vi "Acquire Data using 5772 without DRAM_sim.vi"() -> ()   [LabVIEW 2011]
uses:
  <vilib>/Platform/TimedLoop/XDataNode/timing_clust.ctl
  <vilib>/Platform/TimedLoop/XDataNode/nitl_modes.ctl
  <vilib>/Platform/TimedLoop/XDataNode/wakeup.ctl
  Channel Data/Data from Channel 0 and Channel 1.vi
  <instrlib>/FlexRIO/Libraries/Acquisition Engine/FPGA/Implementation/acqEngineNRecordStateMachine.vi
  <vilib>/rvi/FIFO/Fifo_Resource/nirvififoEmulationSetSize.vi
  <vilib>/rvi/DataTransferAndStorage/Container/Common/niFpgaContainerGetUniqueNameForEmu.vi
  <instrlib>/FlexRIO/Libraries/Acquisition Engine/FPGA/Implementation/Pack 8-I16 As U128.vi
  <instrlib>/FlexRIO/Libraries/Host Transfer/FPGA/Implementation/Write to Host-Bound Domain (128-bit to 64-bit).vi
  <vilib>/Platform/TimedLoop/XDataNode/XDataNode.xnode
  <vilib>/rvi/FXPMathLib/basic elements/FxpDiscreteDelay/XNode/nifxpmath_DiscreteDelay.xnode
  <vilib>/rvi/DataTransferAndStorage/Container/XNode/niFpgaContainer.xnode
  <vilib>/rvi/FIFO/Fifo_Resource/nirvififoEmulationWrite.vi
  <vilib>/rvi/FIFO/Fifo_Resource/nirvififoEmulationRead.vi
  <vilib>/Platform/TimedLoop/XDataNode/XDNodeRunTimeDep.lvlib
  <vilib>/eio/EIONode/EIONode.xnode
  <instrlib>/FlexRIO/Libraries/Acquisition Engine/Acquisition Engine.lvlib
  <vilib>/rvi/eio/common/nirviEmuTemplateMethod_errors.vi
  <instrlib>/FlexRIO/Libraries/Host Transfer/Host Transfer.lvlib
panel:
  out "Channel 1":i16(graph)
  out "Channel 0":i16(graph)
  out "NumSamplestoHost":u32
  out "NumSamplesAcquired":u32
  out "Host FIFO Timed Out?":bool
  in  "Host Trigger":bool=TRUE
  in  "Trigger Type":T1(ring)=enum."Software Trigger"
  out "IO Module\\Initialization Done":bool
  in  "acq.Post Trig":u32=10
  in  "acq.Pre Trig":u32=2 min=2 step=1
  in  "acq.Record Count":u32=1
  in  "acq.Initiate":bool=TRUE
  # "Digitial Trigger Input:\nPXI_Trig0 or DIO 0 on CB Front Panel"
  # "Interactive Mode Instructions\n1) Run the Emulation Mode VI for Stimulus\n1) Click on acq.Initiate, First to False and Then to True\n2) Click on Host Trigger"
  # "Trigger Selection"
  # "Acquisition Engine"
  # "Status"
  # "Record Retrieval"
  # "Memory Configuration"
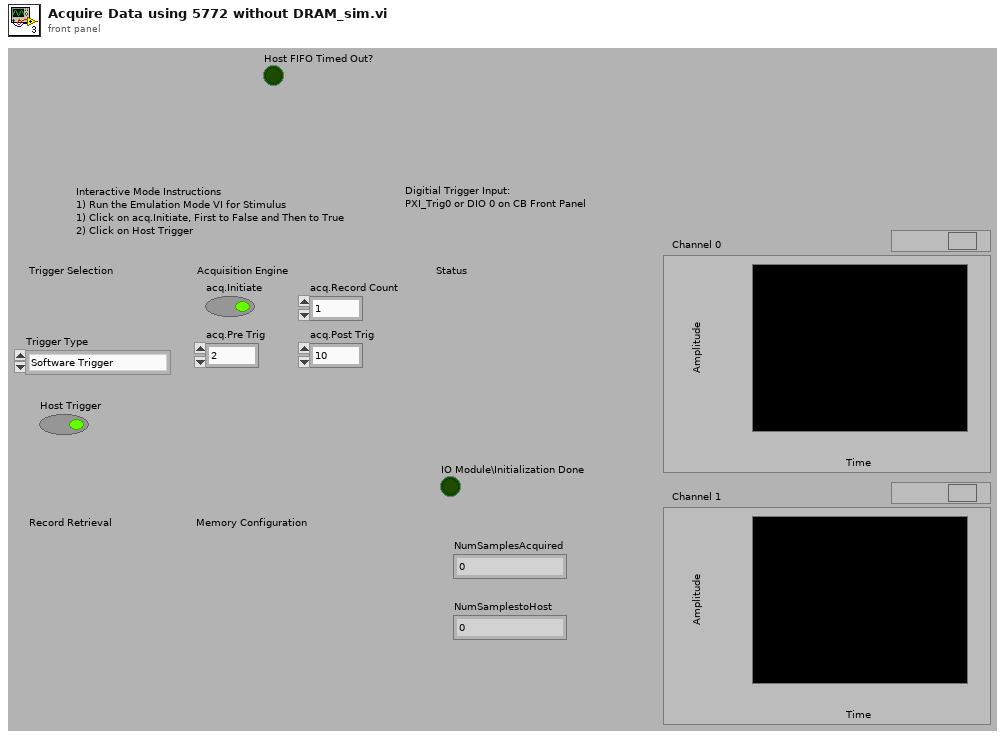
[diagram p1: front panel]
types:
  T1 = enum8{"Immediate Trigger", "Software Trigger", "External Digital Trigger", "Analog Trigger"}
  T2 = typedef "XDNodeRunTimeDep.lvlib/timing_clust.ctl" = cluster{"Expected End [f-1]":u64, "Actual End [f-1]":u64, "Finished Late? [f-1]":bool, "Expected End [i-1]":u64, "Actual End [i-1]":u64, "Finished Late? [i-1]":bool, "Expected Start [i]":u64, "Actual Start [i]":u64, "Expected Start [f]":u64, "Actual Start [f]":u64, "Source Name":string, "Structure Name":string, "Period":i64, "Deadline":i64, "Offset":i64, "Start":i64, "Priority":i32, "Timeout":i32, "Mode":T3, "Wakeup Reason":T4, "Error":errorcluster, "Source Type":string, "Secondary Source Type":string, "Global End Time":u64, "Global Start Time":u64, "Frame Duration":u64, "Iteration Duration":u64, "Assigned CPU":i32, "I/O Scan Engine Mode":u32}
  T3 = typedef "XDNodeRunTimeDep.lvlib/nitl_modes.ctl" = enum32{"No Change", "Process missed periods, maintain original phase", "Discard missed periods, maintain original phase", "Process missed periods, ignore original phase", "Discard missed periods, ignore original phase"}
  T4 = typedef "XDNodeRunTimeDep.lvlib/wakeup.ctl" = enum32{"Normal", "Aborted", "Asynchronous wakeup", "Timing source error", "Timed loop error", "Timeout"}
  T5 = typedef "Memory.lvlib/U128.ctl" = u8[]
  T6 = typedef "acqEngineStates v1.ctl" = cluster{"Triggered":bool, "TrigArmed":bool, "RdyForArm":bool, "Reserved":bool}
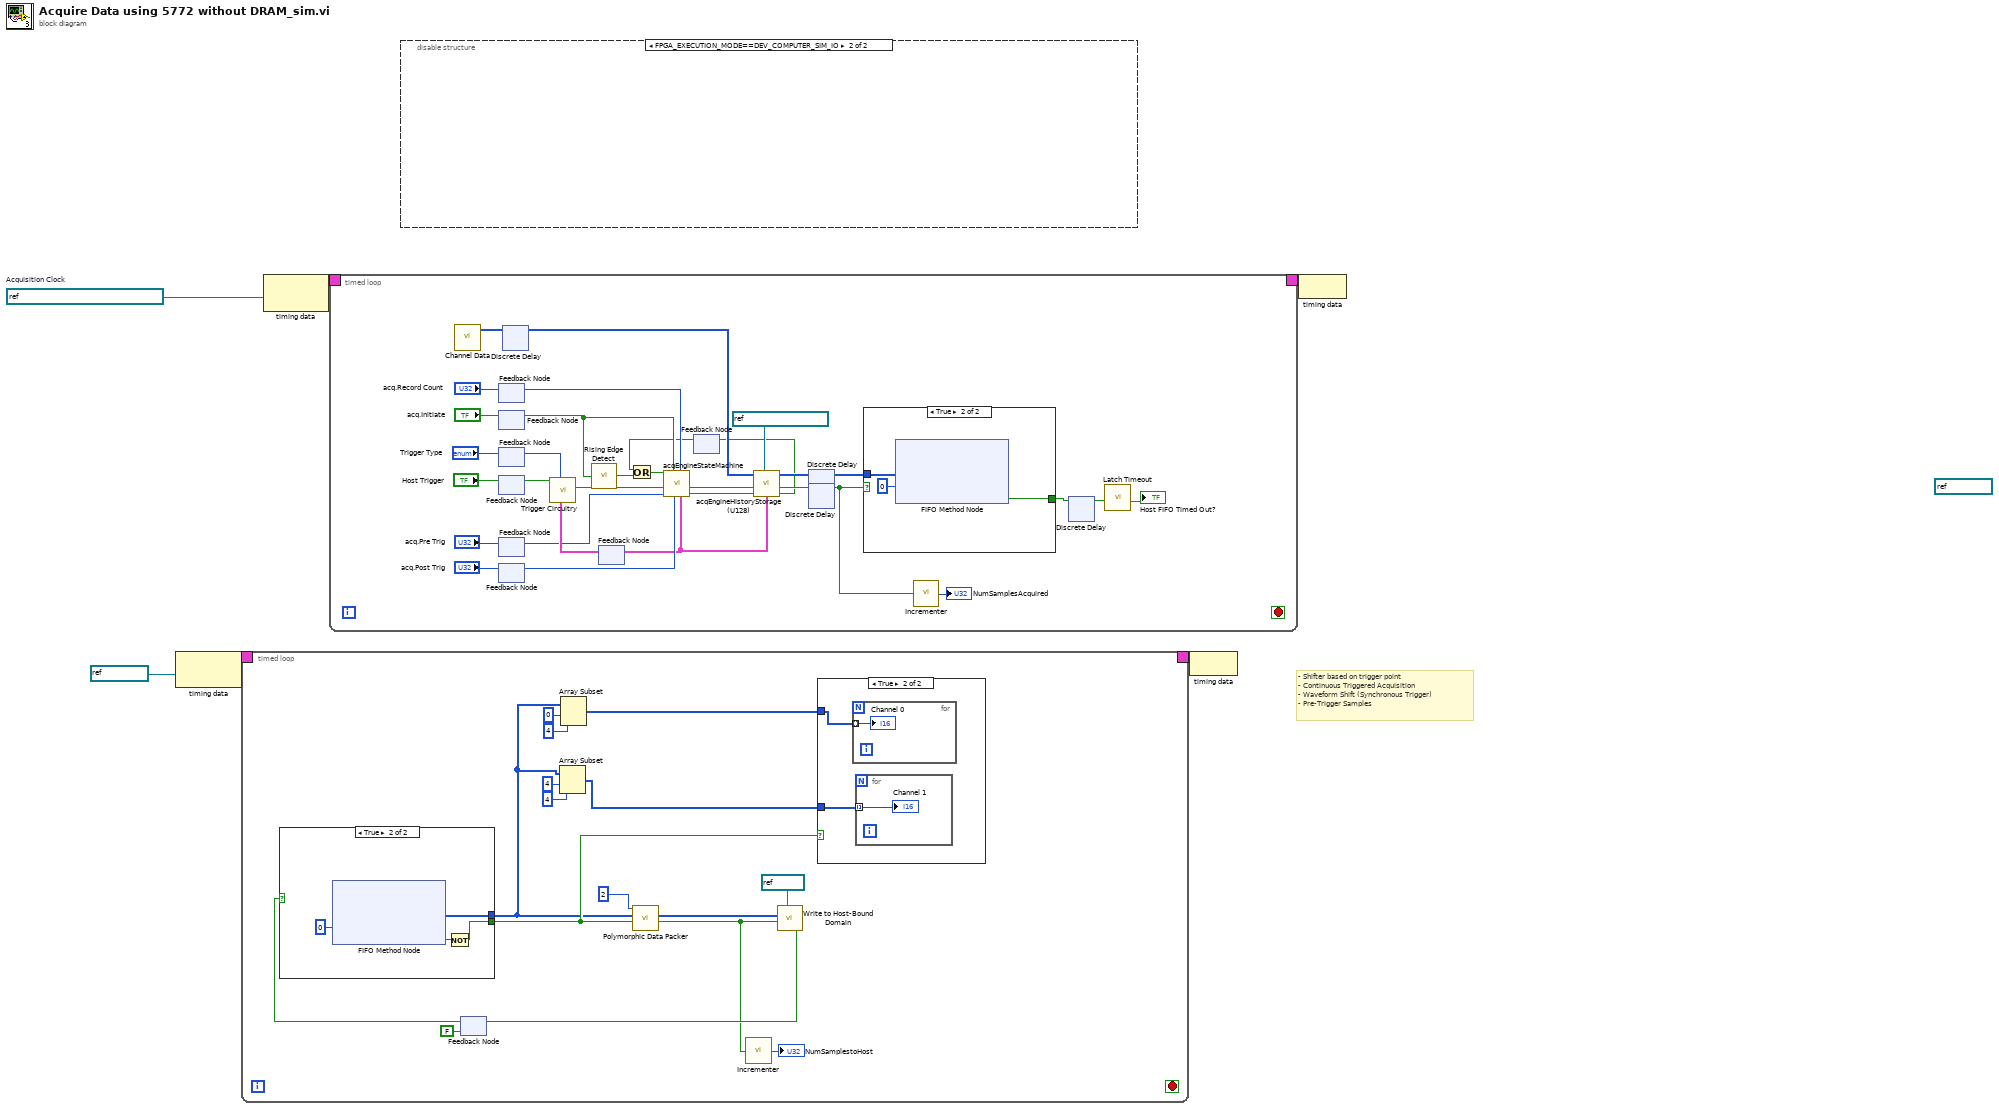
[diagram p0: block diagram]
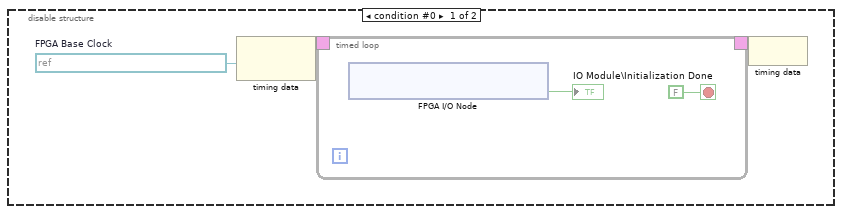
[diagram p2: hidden frame]
diagram:
  (unwired) refnum<k21> "To Host" ("FIFO In")
  w4 = refnum<k21> "IO Module Clock 0"  # Acquisition Clock
  # "- Shifter based on trigger point\n- Continuous Triggered Acquisition\n- Waveform Shift (Synchronous Trigger)\n- Pre-Trigger Samples"
  n1 = node-c288(refnum<k21> "125MHz" ("Source Name")) -> (w3:T2)
  n2 = timed-loop {
    timing: w3 -> [_]
    timing-out: [_] -> w2
    stop <- _ stop-if-true
    n3 = feedback #1(FALSE ("Ready For Input")) -> (w20:bool)
    n4 = case shown="True" w20 {
      tunnel: [_ w29] -> w8
      tunnel: [_ w27] -> w14
      frame False {
      }
      frame True {
        n5 = xnode ("FIFO Method Node")("Timeout"=0) -> ("Element"=w29:i16[], "Timed Out?"=w28:bool)  [unwired: 1 in, 1 out]
        n6 = Not(x=w28) -> (.not. x?=w27:bool)
      }
    }
    n7 = Array Subset(array=w8, index=4, length=4) -> (w7:i16[])
    n8 = Array Subset(array=w8, index=0, length=4) -> (w11:i16[])
    n9 = call-poly <instrlib>:"Polymorphic Data Packer.vi"("enable"=w14, "data"=w8, "Channels Per Unit"=u8 2) -> ("validOut"=w15:bool, "i16 as i128"=w16:T5)  [unwired: 4 in, 3 out]
    n10 = call <userlib>:"Incrementer.vi"("INC?"=w15) -> ("count"=→"NumSamplestoHost":u32)  [unwired: 4 in]
    n11 = call-poly <instrlib>:"Write to Host-Bound Domain.vi"("data"=w16, "valid"=w15, "FIFO Out"=refnum<k21> "FIFO") -> ("Ready For Input"=w21:bool)  [unwired: 4 in]
    n12 = feedback-in #1(w21) -> ()
    n13 = case shown="True" w14 {
      tunnel: w11 -> [_ w24]
      tunnel: w7 -> [_ w23]
      frame False {
      }
      frame True {
        n14 = for {
          tunnel: w24 -> [w26] mode=indexing
          "Channel 0" <- w26
        }
        n15 = for {
          tunnel: w23 -> [w25] mode=indexing
          "Channel 1" <- w25
        }
      }
    }
  }
  n16 = node-c288(w4) -> (w6:T2)
  n17 = timed-loop {
    timing: w6 -> [_]
    timing-out: [_] -> w5
    stop <- _ stop-if-true
    n18 = call-poly "Channel Data.vi"() -> ("Channels Data"=w53:i16[])  [unwired: 11 in]
    n19 = feedback-in #2("acq.Record Count") -> ()
    n20 = feedback #2() -> (w57:u32)  [unwired: 1 in]
    n21 = feedback-in #3("acq.Initiate") -> ()
    n22 = feedback #3() -> (w37:bool)  [unwired: 1 in]
    n23 = feedback #4() -> (w55:T1)  [unwired: 1 in]
    n24 = feedback-in #4("Trigger Type") -> ()
    n25 = feedback-in #5("Host Trigger") -> ()
    n26 = feedback #5() -> (w54:bool)  [unwired: 1 in]
    n27 = feedback-in #6("acq.Pre Trig") -> ()
    n28 = feedback #6() -> (w52:u32)  [unwired: 1 in]
    n29 = feedback-in #7("acq.Post Trig") -> ()
    n30 = feedback #7() -> (w51:u32)  [unwired: 1 in]
    n31 = xnode "Discrete Delay"("D"=w53) -> ("Q"=w47:i16[])
    n32 = call <userlib>:"Rising Edge Detect.vi"("signal"=w37) -> ("edge detected"=w35:bool)  [unwired: 14 in]
    n33 = feedback #8() -> (w59:T6)  [unwired: 1 in]
    n34 = call <userlib>:"Trigger Circuitry.vi"("State Machine State"=w59, "Trigger Type"=w55, "Software Trigger from Host"=w54) -> ("Trigger Out"=w60:bool)  [unwired: 7 in, 1 out]
    n35 = feedback #9() -> (w33:bool)  [unwired: 1 in]
    n36 = Or(x=w33, y=w35) -> (x .or. y?=w36:bool)
    n37 = call-poly <instrlib>:"acqEngineStateMachine.vi"("acq.Record Count"=w57, "acq.Post Trig"=w51, "acq.Initiate"=w37, "acq.Pre Trig"=w52, "Trig"=w60, "StartTrig"=w36) -> ("PostTrigComplete"=w48:bool, "AcqInProgress"=w49:bool, "states"=w50:T6)  [unwired: 3 in]
    n38 = feedback-in #8(w50) -> ()
    n39 = call "acqEngineHistoryStorage (U128).vi"("FIFO Out"=refnum<k21> "HistoryFIFOU128", "PostTrigComplete"=w48, "AcqInProgress"=w49, "states"=w50, "Input Data"=w47) -> ("flushed"=w34:bool, "valid"=w44:bool, "Output Data"=w45:i16[])  [unwired: 4 in]
    n40 = feedback-in #9(w34) -> ()
    n41 = xnode "Discrete Delay"("D"=w45) -> ("Q"=w40:i16[])
    n42 = xnode "Discrete Delay"("D"=w44) -> ("Q"=w39:bool)
    n43 = case shown="True" w39 {
      tunnel: w40 -> [_ w67]
      tunnel: [_ w65] -> w41
      frame False {
      }
      frame True {
        n44 = xnode ("FIFO Method Node")("Element"=w67, "Timeout"=0) -> ("Timed Out?"=w65:bool)  [unwired: 1 in, 1 out]
      }
    }
    n45 = call <userlib>:"Incrementer.vi"("INC?"=w39) -> ("count"=→"NumSamplesAcquired":u32)  [unwired: 4 in]
    n46 = xnode "Discrete Delay"("D"=w41) -> ("Q"=w42:bool)
    n47 = call <userlib>:"Latch Timeout.vi"("Timeout?"=w42) -> ("Ever Timed Out?"=→"Host FIFO Timed Out?":bool)  [unwired: 10 in]
  }
  n48 = disable-structure shown="FPGA_EXECUTION_MODE==DEV_COMPUTER_SIM_IO" {
    frame condition #0 {
      w70 = refnum<k21> "40 MHz Onboard Clock"  # FPGA Base Clock
      n49 = node-c288(w70) -> (w72:T2)
      n50 = timed-loop {
        timing: w72 -> [_]
        timing-out: [_] -> w71
        stop <- FALSE stop-if-true
        n51 = xnode "FPGA I/O Node"() -> ("IO Module\\Initialization Done"=→"IO Module\\Initialization Done":bool)  [unwired: 1 in, 1 out]
      }
      n52 = node-c288(w71) -> ()
    }
    frame condition #1 (active) {
    }
  }
  n53 = node-c288(w2) -> ()
  n54 = node-c288(w5) -> ()
